vi "HFRR ADV v025 new software.vi"() -> ()   [LabVIEW 2025] (continued)
        n322 = event-data() -> ()  [unwired: 1 in, 6 out]
        n323 = Unbundle By Name("Password 3") -> ("Service Password"=w406:string)
        n324 = call <vilib>:"Trim Whitespace.vi"("string"=w406) -> ("trimmed string"=w404:string)  [unwired: 1 in]
        n325 = Equal?(x=w404, y="Service@123") -> (x = y?=w405:bool)
        n326 = case shown="False" w405 {
          selector: w405 -> [w409 w411]
          frame False {
            n327 = local write "Service Password enable"(w409) -> ()
            n328 = property on="Service Password Log" class="Str"("Visible"=TRUE) -> ()  [unwired: 2 in, 2 out]
          }
          frame True {
            n329 = property on="Service Password Log" class="Str"("Visible"=FALSE) -> ()  [unwired: 2 in, 2 out]
            "Service Password enable" <- w411
          }
        }
      }
      event "Sign In": Value Change {
        w413 = FALSE ("Visible")
        n330 = event-data() -> ()  [unwired: 1 in, 6 out]
        n331 = property on="About" class="Clust (strict)"("Visible"=w413) -> ()  [unwired: 2 in, 2 out]
        n332 = property on="Password 3" class="Clust (strict)"("Visible"=w413) -> ()  [unwired: 2 in, 2 out]
        n333 = property on="Service Password Log" class="Str"("Visible"=FALSE) -> ()  [unwired: 2 in, 2 out]
      }
      event "Info": Value Change {
        n334 = event-data() -> ()  [unwired: 1 in, 6 out]
        n335 = local read "Info"() -> (w415:bool)
        n336 = case shown="False" w415 {
          frame False {
            n337 = property on="About" class="Clust (strict)"("Visible"=FALSE) -> ()  [unwired: 2 in, 2 out]
          }
          frame True {
            n338 = property on="About" class="Clust (strict)"("Visible"=TRUE) -> ()  [unwired: 2 in, 2 out]
          }
        }
      }
      event "Calibration": Value Change {
        n339 = event-data() -> ()  [unwired: 1 in, 6 out]
        n340 = local read "Calibration"() -> (w419:bool)
        n341 = case shown="False" w419 {
          frame False {
            n342 = property on="Calibration 2" class="TabCtl (strict)"("Visible"=FALSE) -> ()  [unwired: 2 in, 2 out]
            n343 = local write "Cal Password"("" ("Cal Password")) -> ()
          }
          frame True {
            n344 = property on="Calibration 2" class="TabCtl (strict)"("Visible"=TRUE) -> ()  [unwired: 2 in, 2 out]
            n345 = local write "Cal Password"("" ("Cal Password")) -> ()
          }
        }
        n346 = property on="Wrong Password" class="Str"("Visible"=FALSE) -> ()  [unwired: 2 in, 2 out]
      }
      event "Cal Password": Value Change {
        n347 = event-data() -> ()  [unwired: 1 in, 6 out]
        n348 = local read "Cal Password"() -> (w427:string)
        n349 = call <vilib>:"Trim Whitespace.vi"("string"=w427) -> ("trimmed string"=w426:string)  [unwired: 1 in]
        n350 = Equal?(x=w426, y="Cal@321") -> (x = y?=w424:bool)
        n351 = case shown="True" w424 {
          frame False {
            n352 = property on="Wrong Password" class="Str"("Visible"=TRUE) -> ()  [unwired: 2 in, 2 out]
          }
          frame True {
            n353 = property on="Wrong Password" class="Str"("Visible"=FALSE) -> ()  [unwired: 2 in, 2 out]
            n354 = local write "Main Tab"(T2."About" ("Main Tab")) -> ()
            n355 = local write "Cal Password"("" ("Cal Password")) -> ()
            n356 = local write "Main Dashboard Buttons"(T1."About" ("Main Dashboard Buttons")) -> ()
            n357 = property on="Calibration 2" class="TabCtl (strict)"("Visible"=FALSE) -> ()  [unwired: 2 in, 2 out]
            n358 = local write "Calibration"(FALSE ("Calibration")) -> ()
          }
        }
      }
      event "Calibration Selection": Value Change {
        n359 = event-data() -> ()  [unwired: 1 in, 6 out]
        n360 = local read "Calibration Selection"() -> (w436:T8)
        n361 = case shown="\"Stroke Calibration\"" w436 {
          tunnel: [T7."Stroke" ("Main Calibration Tab") T7."Friction" ("Main Calibration Tab") T7."Main" ("Main Calibration Tab") T7."Temperature" ("Main Calibration Tab")] -> w435
          frame "Stroke Calibration" {
          }
          frame "Friction Force Calibration" {
          }
          frame Default {
          }
          frame "Temperature Calibration" {
          }
        }
        n362 = local write "Main Calibration Tab"(w435) -> ()
      }
      event "Back Stroke": Value Change {
        n363 = event-data() -> ()  [unwired: 1 in, 6 out]
        n364 = local write "Main Stroke Tab"(T9."Step 1" ("Main Stroke Tab")) -> ()
        n365 = local write "Main Calibration Tab"(T7."Main" ("Main Calibration Tab")) -> ()
        n366 = local write "Back Stroke"(FALSE ("Back Stroke")) -> ()
      }
      event "Step 2 Back": Value Change {
        n367 = event-data() -> ()  [unwired: 1 in, 6 out]
        n368 = local write "Main Stroke Tab"(T9."Step 1" ("Main Stroke Tab")) -> ()
        n369 = local write "Step 2 Back"(FALSE ("Back Stroke")) -> ()
      }
      event "Step 3 Back": Value Change {
        n370 = event-data() -> ()  [unwired: 1 in, 6 out]
        n371 = local write "Main Stroke Tab"(T9."Step 2" ("Main Stroke Tab")) -> ()
        n372 = local write "Step 3 Back"(FALSE ("Back Stroke")) -> ()
      }
      event "Step 4 Back": Value Change {
        n373 = event-data() -> ()  [unwired: 1 in, 6 out]
        n374 = local write "Main Stroke Tab"(T9."Step 3" ("Main Stroke Tab")) -> ()
        n375 = local write "Step 4 Back"(FALSE ("Back Stroke")) -> ()
      }
      event "Step 5 Back": Value Change {
        n376 = event-data() -> ()  [unwired: 1 in, 6 out]
        n377 = local write "Main Stroke Tab"(T9."Step 4" ("Main Stroke Tab")) -> ()
        n378 = local write "Step 5 Back"(FALSE ("Back Stroke")) -> ()
      }
      event "Step 6 Back": Value Change {
        n379 = event-data() -> ()  [unwired: 1 in, 6 out]
        n380 = local write "Main Stroke Tab"(T9."Step 5" ("Main Stroke Tab")) -> ()
        n381 = local write "Step 6 Back"(FALSE ("Back Stroke")) -> ()
      }
      event "Back Stroke step 7": Value Change {
        n382 = event-data() -> ()  [unwired: 1 in, 6 out]
        n383 = local write "Main Stroke Tab"(T9."Step 6" ("Main Stroke Tab")) -> ()
        n384 = local write "Back Stroke step 7"(FALSE ("Back Stroke")) -> ()
      }
      event "Back Stroke step 8": Value Change {
        n385 = event-data() -> ()  [unwired: 1 in, 6 out]
        n386 = local write "Main Stroke Tab"(T9."Step 7" ("Main Stroke Tab")) -> ()
        n387 = local write "Back Stroke step 8"(FALSE ("Back Stroke")) -> ()
      }
      event "Back Stroke 8": Value Change {
        n388 = event-data() -> ()  [unwired: 1 in, 6 out]
        n389 = local write "MOVE CARRIAGE TO"(0.2 ("MOVE CARRIAGE TO")) -> ()
        n390 = local write "Main Stroke Tab"(T9."Step 1" ("Main Stroke Tab")) -> ()
        n391 = local write "Back Stroke 8"(FALSE ("Back Stroke 8")) -> ()
      }
      event "Continue Stroke": Value Change {
        n392 = event-data() -> ()  [unwired: 1 in, 6 out]
        n393 = local write "Main Stroke Tab"(T9."Step 2" ("Main Stroke Tab")) -> ()
        n394 = local write "Continue Stroke"(FALSE ("Continue Stroke")) -> ()
      }
      event "Continue Stroke step 2": Value Change {
        n395 = event-data() -> ()  [unwired: 1 in, 6 out]
        n396 = local write "Main Stroke Tab"(T9."Step 3" ("Main Stroke Tab")) -> ()
        n397 = local write "Continue Stroke step 2"(FALSE ("Continue Stroke")) -> ()
      }
      event "Continue Stroke step 3": Value Change {
        n398 = event-data() -> ()  [unwired: 1 in, 6 out]
        n399 = local write "Main Stroke Tab"(T9."Step 4" ("Main Stroke Tab")) -> ()
        n400 = local write "Continue Stroke step 3"(FALSE ("Continue Stroke")) -> ()
      }
      event "Continue Stroke step 4": Value Change {
        n401 = event-data() -> ()  [unwired: 1 in, 6 out]
        n402 = local write "Main Stroke Tab"(T9."Step 5" ("Main Stroke Tab")) -> ()
        n403 = local write "Continue Stroke step 4"(FALSE ("Continue Stroke")) -> ()
      }
      event "Continue Stroke step 5": Value Change {
        n404 = event-data() -> ()  [unwired: 1 in, 6 out]
        n405 = local write "Main Stroke Tab"(T9."Step 6" ("Main Stroke Tab")) -> ()
        n406 = local write "Continue Stroke step 5"(FALSE ("Continue Stroke")) -> ()
      }
      event "Continue Stroke step 6": Value Change {
        n407 = event-data() -> ()  [unwired: 1 in, 6 out]
        n408 = local write "Main Stroke Tab"(T9."Step 7" ("Main Stroke Tab")) -> ()
        n409 = local write "Continue Stroke step 6"(FALSE ("Continue Stroke")) -> ()
      }
      event "Continue Stroke step 7": Value Change {
        w475 = FALSE ("0.2mm")
        n410 = event-data() -> ()  [unwired: 1 in, 6 out]
        n411 = local write "0.4 mm"(w475) -> ()
        n412 = local write "0.6 mm"(w475) -> ()
        n413 = local write "1.0 mm"(w475) -> ()
        n414 = local write "1.2 mm"(w475) -> ()
        n415 = local write "0.2 2"(w475) -> ()
        n416 = local write "0.4 2"(w475) -> ()
        n417 = local write "0.6 2"(w475) -> ()
        n418 = local write "0.8 2"(w475) -> ()
        n419 = local write "1.0 2"(w475) -> ()
        n420 = local write "1.2"(w475) -> ()
        n421 = local write "0.2mm"(w475) -> ()
        n422 = local write "0.8mm"(w475) -> ()
        n423 = local write "Main Stroke Tab"(T9."Step 8" ("Main Stroke Tab")) -> ()
        n424 = local write "Continue Stroke step 7"(FALSE ("Continue Stroke")) -> ()
        n425 = local write "Stroke Test Complete"(T10."Test Progress" ("Stroke Test Complete")) -> ()
        "Position Measurment Temp" <- 0.0 ("Position Measurment Temp")
        "Calibration Tare" <- TRUE ("Calibration Tare")
        "MOVE CARRIAGE TO" <- 0.2 ("MOVE CARRIAGE TO")
      }
      event "Continue Stroke step 8": Value Change {
        n426 = event-data() -> ()  [unwired: 1 in, 6 out]
        n427 = local read "LVDT STROKE  Calibration"() -> (w480:dbl)
        n428 = local read "Position Measurment Temp"() -> (w481:dbl)
        n429 = case shown="7" w481 {
          selector: w481 -> [w486 w491 w496 w501 w506 w510 w513 w514]
          tunnel: w480 -> [w482 w487 w492 w497 w502 w507 _ _]
          frame 0, Default {
            w484 = TRUE ("0.2mm")
            n430 = Increment(x=w486) -> (x+1=w485:i32)
            n431 = local write "Position Measurment Temp"(w485) -> ()
            n432 = local write "0.2mm"(w484) -> ()
            n433 = local write "0.2 2"(w484) -> ()
            n434 = local write "MOVE CARRIAGE TO"(0.4 ("MOVE CARRIAGE TO")) -> ()
            "Calibration 0.2" <- w482
          }
          frame 1 {
            w489 = TRUE ("0.4 mm")
            n435 = Increment(x=w491) -> (x+1=w490:i32)
            n436 = local write "Calibration 0.4"(w487) -> ()
            n437 = local write "Position Measurment Temp"(w490) -> ()
            n438 = local write "0.4 mm"(w489) -> ()
            n439 = local write "MOVE CARRIAGE TO"(0.6 ("MOVE CARRIAGE TO")) -> ()
            n440 = local write "0.4 2"(w489) -> ()
          }
          frame 2 {
            w494 = TRUE ("0.6 mm")
            n441 = Increment(x=w496) -> (x+1=w495:i32)
            n442 = local write "Calibration 0.6"(w492) -> ()
            n443 = local write "Position Measurment Temp"(w495) -> ()
            n444 = local write "0.6 2"(w494) -> ()
            n445 = local write "0.6 mm"(w494) -> ()
            n446 = local write "MOVE CARRIAGE TO"(0.8 ("MOVE CARRIAGE TO")) -> ()
          }
          frame 3 {
            w498 = TRUE ("0.6 mm")
            n447 = Increment(x=w501) -> (x+1=w500:i32)
            n448 = local write "Position Measurment Temp"(w500) -> ()
            n449 = local write "MOVE CARRIAGE TO"(1.0 ("MOVE CARRIAGE TO")) -> ()
            n450 = local write "0.8mm"(w498) -> ()
            n451 = local write "0.8 2"(w498) -> ()
            "Calibration 0.8" <- w497
          }
          frame 4 {
            w503 = TRUE ("0.6 mm")
            n452 = Increment(x=w506) -> (x+1=w505:i32)
            n453 = local write "Position Measurment Temp"(w505) -> ()
            n454 = local write "MOVE CARRIAGE TO"(1.2 ("MOVE CARRIAGE TO")) -> ()
            n455 = local write "1.0 mm"(w503) -> ()
            n456 = local write "1.0 2"(w503) -> ()
            "Calibration 1.0" <- w502
          }
          frame 5 {
            w508 = TRUE ("0.6 mm")
            n457 = Increment(x=w510) -> (x+1=w509:i32)
            n458 = local write "Position Measurment Temp"(w509) -> ()
            n459 = local write "1.2 mm"(w508) -> ()
            n460 = local write "1.2"(w508) -> ()
            "Calibration 1.2" <- w507
          }
          frame 6 {
            n461 = Increment(x=w513) -> (x+1=w512:i32)
            n462 = local write "Position Measurment Temp"(w512) -> ()
            n463 = local write "Stroke Test Complete"(T10."Stroke Points Completed" ("Stroke Test Complete")) -> ()
          }
          frame 7 {
            n464 = stacked-sequence {
              tunnel: w514 -> [w515 _ _]
              frame #0 {
                n465 = Increment(x=w515) -> (x+1=w516:i32)
                n466 = local write "Main Stroke Tab"(T9."Step 9" ("Main Stroke Tab")) -> ()
                n467 = local write "Position Measurment Temp"(w516) -> ()
                n468 = Insert Into Array(array=dbl[] [], new element #1=0.2 ("new element/subarray"), new element #2=0.4 ("new element/subarray"), new element #3=0.6 ("new element/subarray"), new element #4=0.8 ("new element/subarray"), new element #5=1.0 ("new element/subarray"), new element #6=1.2 ("new element/subarray")) -> (→"1D stroke":dbl[])  [unwired: 1 in]
                n469 = local read "Calibration 0.2"() -> (w523:dbl)
                n470 = local read "Calibration 0.4"() -> (w522:dbl)
                n471 = local read "Calibration 0.6"() -> (w521:dbl)
                n472 = local read "Calibration 0.8"() -> (w520:dbl)
                n473 = local read "Calibration 1.0"() -> (w519:dbl)
                n474 = local read "Calibration 1.2"() -> (w518:dbl)
                n475 = Insert Into Array(array=dbl[] [], new element #1=w523, new element #2=w522, new element #3=w521, new element #4=w520, new element #5=w519, new element #6=w518) -> (→"Calibrated Voltage Value":dbl[])  [unwired: 1 in]
              }
              frame #1 {
                n476 = local read "calibration values"() -> (w546:dbl[])
                n477 = local read "Calibrated Voltage Value"() -> (w548:dbl[])
                n478 = Index Array(array=w546, index #1=1 ("index"), index #2=3 ("index"), index #3=5 ("index"), index #4=7 ("index"), index #5=9 ("index"), index #6=11 ("index")) -> (element #1=w539:dbl, element #2=w538:dbl, element #3=w537:dbl, element #4=w536:dbl, element #5=w535:dbl, element #6=w534:dbl)
                n479 = local read "1D stroke"() -> (w549:dbl[])
                n480 = for {
                  tunnel: [w558] -> w547 mode=indexing
                  tunnel: w549 -> [w557] mode=indexing
                  tunnel: w548 -> [w556] mode=indexing
                  tunnel: w539 -> [w555]
                  tunnel: w538 -> [w554]
                  tunnel: w537 -> [w553]
                  tunnel: w536 -> [w552]
                  tunnel: w535 -> [w551]
                  tunnel: w534 -> [w550]
                  n481 = formula code="if (stroke == 0.2)\n{\n    if ((voltage >= REF_02 * 0.985) && (voltage <= REF_02 * 1.015))\n        status = 1;\n    else\n        status = 0;\n}\nelse if (stroke == 0.4)\n{\n    if ((voltage >= REF_04 * 0.985) && (voltage <= REF_04 * 1.015))\n        status = 1;\n    else\n        status = 0;\n}\nelse if (stroke == 0.6)\n{\n    if ((voltage >= REF_06 * 0.985) && (voltage <= REF_06 * 1.015))\n        status = 1;\n    else\n        status = 0;\n}\nelse if (stroke == 0.8)\n{\n    if ((voltage >= REF_08 * 0.985) && (voltage <= REF_08 * 1.015))\n        status = 1;\n    else\n        status = 0;\n}\nelse if (stroke == 1.0)\n{\n    if ((voltage >= REF_10 * 0.985) && (voltage <= REF_10 * 1.015))\n        status = 1;\n    else\n        status = 0;\n}\nelse if (stroke == 1.2)\n{\n    if ((voltage >= REF_12 * 0.985) && (voltage <= REF_12 * 1.015))\n        status = 1;\n    else\n        status = 0;\n}\nelse\n{\n    status = 0;\n}"("stroke"=w557, "voltage"=w556, "REF_02"=w555, "REF_04"=w554, "REF_06"=w553, "REF_08"=w552, "REF_10"=w551, "REF_12"=w550) -> ("status"=w558:dbl)
                }
                "Status" <- w547
              }
              frame #2 {
                w565 = 1.0
                n482 = local read "Status"() -> (w572:dbl[])
                n483 = Index Array(array=w572) -> (element #1=w571:dbl, element #2=w570:dbl, element #3=w569:dbl, element #4=w568:dbl, element #5=w567:dbl, element #6=w566:dbl)  [unwired: 6 in]
                n484 = Equal?(x=w570, y=w565) -> (x = y?=w563:bool)
                n485 = Equal?(x=w569, y=w565) -> (x = y?=w562:bool)
                n486 = Equal?(x=w568, y=w565) -> (x = y?=w561:bool)
                n487 = Equal?(x=w567, y=w565) -> (x = y?=w560:bool)
                n488 = Equal?(x=w566, y=w565) -> (x = y?=w559:bool)
                n489 = Equal?(x=w571, y=w565) -> (x = y?=w564:bool)
                n490 = case shown="True" w564 {
                  selector: w564 -> [w583 w584]
                  frame True {
                    n491 = local write "Point 1 - 0.2 mm"(w583) -> ()
                    n492 = property on="Point 1 - 0.2 mm" class="Bool"("Caption.Visible"=w583) -> ()  [unwired: 2 in, 2 out]
                  }
                  frame False {
                    n493 = local write "Point 1 - 0.2 mm"(w584) -> ()
                    n494 = property on="Point 1 - 0.2 mm" class="Bool"("Caption.Visible"=w584) -> ()  [unwired: 2 in, 2 out]
                  }
                }
                n495 = case shown="True" w563 {
                  selector: w563 -> [w581 w582]
                  frame True {
                    n496 = local write "Point 2 - 0.4 mm"(w581) -> ()
                    n497 = property on="Point 2 - 0.4 mm" class="Bool"("Caption.Visible"=w581) -> ()  [unwired: 2 in, 2 out]
                  }
                  frame False {
                    n498 = local write "Point 2 - 0.4 mm"(w582) -> ()
                    n499 = property on="Point 2 - 0.4 mm" class="Bool"("Caption.Visible"=w582) -> ()  [unwired: 2 in, 2 out]
                  }
                }
                n500 = case shown="True" w560 {
                  selector: w560 -> [w575 w576]
                  frame True {
                    n501 = local write "Point 5 - 1.0 mm"(w575) -> ()
                    n502 = property on="Point 5 - 1.0 mm" class="Bool"("Caption.Visible"=w575) -> ()  [unwired: 2 in, 2 out]
                  }
                  frame False {
                    n503 = local write "Point 5 - 1.0 mm"(w576) -> ()
                    n504 = property on="Point 5 - 1.0 mm" class="Bool"("Caption.Visible"=w576) -> ()  [unwired: 2 in, 2 out]
                  }
                }
                n505 = case shown="True" w562 {
                  selector: w562 -> [w579 w580]
                  frame True {
                    n506 = local write "Point 3 - 0.6 mm"(w579) -> ()
                    n507 = property on="Point 3 - 0.6 mm" class="Bool"("Caption.Visible"=w579) -> ()  [unwired: 2 in, 2 out]
                  }
                  frame False {
                    n508 = local write "Point 3 - 0.6 mm"(w580) -> ()
                    n509 = property on="Point 3 - 0.6 mm" class="Bool"("Caption.Visible"=w580) -> ()  [unwired: 2 in, 2 out]
                  }
                }
                n510 = case shown="True" w561 {
                  selector: w561 -> [w577 w578]
                  frame True {
                    n511 = local write "Point 4 - 0.8 mm"(w577) -> ()
                    n512 = property on="Point 4 - 0.8 mm" class="Bool"("Caption.Visible"=w577) -> ()  [unwired: 2 in, 2 out]
                  }
                  frame False {
                    n513 = local write "Point 4 - 0.8 mm"(w578) -> ()
                    n514 = property on="Point 4 - 0.8 mm" class="Bool"("Caption.Visible"=w578) -> ()  [unwired: 2 in, 2 out]
                  }
                }
                n515 = case shown="True" w559 {
                  selector: w559 -> [w573 w574]
                  frame True {
                    n516 = local write "Point 6 - 1.2 mm"(w573) -> ()
                    n517 = property on="Point 6 - 1.2 mm" class="Bool"("Caption.Visible"=w573) -> ()  [unwired: 2 in, 2 out]
                  }
                  frame False {
                    n518 = local write "Point 6 - 1.2 mm"(w574) -> ()
                    n519 = property on="Point 6 - 1.2 mm" class="Bool"("Caption.Visible"=w574) -> ()  [unwired: 2 in, 2 out]
                  }
                }
              }
            }
          }
        }
      }
      event "TEMPERATURE STEP Back 1", "TEMPERATURE STEP Back air Temp": Value Change {
        n520 = event-data() -> ()  [unwired: 1 in, 6 out]
        n521 = stacked-sequence {
          frame #0 {
            n522 = local write "Main Calibration Tab"(T7."Main" ("Main Calibration Tab")) -> ()
          }
          frame #1 {
            n523 = Wait (ms)(milliseconds to wait=u32 1000) -> ()  [unwired: 1 out]
          }
          frame #2 {
            n524 = local write "Due Write"("CAL;END" ("Command")) -> ()
          }
          frame #3 {
            n525 = Wait (ms)(milliseconds to wait=u32 2000) -> ()  [unwired: 1 out]
          }
          frame #4 {
            n526 = local write "Due Write"("CAL;END" ("Command")) -> ()
          }
        }
      }
      event "Temperature Continue Step 1": Value Change {
        n527 = event-data() -> ()  [unwired: 1 in, 6 out]
        n528 = stacked-sequence {
          frame #0 {
            n529 = Wait (ms)(milliseconds to wait=u32 1500) -> ()  [unwired: 1 out]
          }
          frame #1 {
            n530 = local write "Due Write"("CAL;START" ("Command")) -> ()
          }
          frame #2 {
            n531 = Wait (ms)(milliseconds to wait=u32 1500) -> ()  [unwired: 1 out]
          }
          frame #3 {
            n532 = local write "Due Write"("CAL;START" ("Command")) -> ()
          }
          frame #4 {
            n533 = Wait (ms)(milliseconds to wait=u32 2000) -> ()  [unwired: 1 out]
          }
          frame #5 {
          }
          frame #6 {
            n534 = Wait (ms)(milliseconds to wait=u32 2000) -> ()  [unwired: 1 out]
          }
          frame #7 {
            # "CAL;A1;<true_T>"
            n535 = local write "Due Write"("CAL;A1;0" ("Command")) -> ()
          }
          frame #8 {
            n536 = local write "Tab Control 4"(T11."Step 2" ("Tab Control 4")) -> ()
          }
        }
      }
      event "Temperature Continue Step air Step 1": Value Change {
        n537 = event-data() -> ()  [unwired: 1 in, 6 out]
        n538 = stacked-sequence {
          frame #0 {
            n539 = Wait (ms)(milliseconds to wait=u32 1500) -> ()  [unwired: 1 out]
          }
          frame #1 {
            n540 = local write "Due Write"("CAL;START" ("Command")) -> ()
          }
          frame #2 {
            n541 = local write "Tab Control 4"(T11."Air Step 2" ("Tab Control 4")) -> ()
            n542 = Wait (ms)(milliseconds to wait=u32 1500) -> ()  [unwired: 1 out]
          }
          frame #3 {
            n543 = local write "Due Write"("CAL;START" ("Command")) -> ()
          }
          frame #4 {
            n544 = Wait (ms)(milliseconds to wait=u32 2000) -> ()  [unwired: 1 out]
          }
          frame #5 {
            # "CAL;A1;<true_T>"
            n545 = local write "Due Write"("CAL;A2;0" ("Command")) -> ()
          }
          frame #6 {
            n546 = Wait (ms)(milliseconds to wait=u32 2000) -> ()  [unwired: 1 out]
          }
          frame #7 {
            # "CAL;A1;<true_T>"
            n547 = local write "Due Write"("CAL;A1;0" ("Command")) -> ()
          }
        }
      }
      event "Temperature Selection": Value Change {
        n548 = event-data() -> ()  [unwired: 1 in, 6 out]
        n549 = local read "Temperature Selection"() -> (w607:enum32{"Air Temperature", "Sample Temperature"})
        n550 = case shown="\"Sample Temperature\"" w607 {
          frame "Air Temperature", Default {
            n551 = local write "Tab Control 4"(T11."Air Step 1" ("Tab Control 4")) -> ()
          }
          frame "Sample Temperature" {
            n552 = local write "Tab Control 4"(T11."Step 1" ("Tab Control 4")) -> ()
          }
        }
      }
      event "Temperature Continue Step 2": Value Change {
        n553 = event-data() -> ()  [unwired: 1 in, 6 out]
        n554 = stacked-sequence {
          frame #0 {
            n555 = stacked-sequence {
              frame #0 {
                n556 = Wait (ms)(milliseconds to wait=u32 1500) -> ()  [unwired: 1 out]
              }
              frame #1 {
                # "CAL;A1;<true_T>"
                n557 = local write "Due Write"("CAL;A1;0" ("Command")) -> ()
              }
              frame #2 {
                n558 = Wait (ms)(milliseconds to wait=u32 1500) -> ()  [unwired: 1 out]
              }
              frame #3 {
                # "CAL;A1;<true_T>"
                n559 = local write "Due Write"("CAL;A1;0" ("Command")) -> ()
              }
              frame #4 {
              }
            }
          }
          frame #1 {
            n560 = local write "Tab Control 4"(T11."Step 3" ("Tab Control 4")) -> ()
          }
        }
      }
      event "Temperature Continue Step 3": Value Change {
        n561 = event-data() -> ()  [unwired: 1 in, 6 out]
        n562 = stacked-sequence {
          frame #0 {
            n563 = stacked-sequence {
              frame #0 {
                n564 = Wait (ms)(milliseconds to wait=u32 1500) -> ()  [unwired: 1 out]
              }
              frame #1 {
              }
              frame #2 {
              }
              frame #3 {
                # "CAL;A1;<true_T>"
                n565 = local write "Due Write"("CAL;A1;60" ("Command")) -> ()
              }
              frame #4 {
                n566 = Wait (ms)(milliseconds to wait=u32 2000) -> ()  [unwired: 1 out]
              }
              frame #5 {
                # "CAL;A1;<true_T>"
                n567 = local write "Due Write"("CAL;A1;60" ("Command")) -> ()
              }
            }
          }
          frame #1 {
            n568 = Wait (ms)(milliseconds to wait=u32 1000) -> ()  [unwired: 1 out]
          }
          frame #2 {
            n569 = local write "Due Write"("CAL;SAVE" ("Command")) -> ()
          }
          frame #3 {
            n570 = Wait (ms)(milliseconds to wait=u32 1000) -> ()  [unwired: 1 out]
          }
          frame #4 {
            n571 = local write "Due Write"("CAL;SAVE" ("Command")) -> ()
          }
          frame #5 {
            n572 = Wait (ms)(milliseconds to wait=u32 1000) -> ()  [unwired: 1 out]
          }
          frame #6 {
            # "CAL;END"
            n573 = local write "Due Write"("CAL;END" ("Command")) -> ()
          }
          frame #7 {
            n574 = Wait (ms)(milliseconds to wait=u32 1000) -> ()  [unwired: 1 out]
          }
          frame #8 {
            # "CAL;END"
            n575 = local write "Due Write"("CAL;END" ("Command")) -> ()
          }
          frame #9 {
            n576 = local write "Main Calibration Tab"(T7."Temperature" ("Main Calibration Tab")) -> ()
            n577 = local write "Tab Control 4"(T11."Main" ("Tab Control 4")) -> ()
          }
        }
      }
      event "Back Stroke step main temperature": Value Change {
        n578 = event-data() -> ()  [unwired: 1 in, 6 out]
        n579 = stacked-sequence {
          frame #0 {
            n580 = Wait (ms)(milliseconds to wait=u32 1000) -> ()  [unwired: 1 out]
          }
          frame #1 {
            # "CAL;END"
            n581 = local write "Due Write"("CAL;END" ("Command")) -> ()
          }
          frame #2 {
            n582 = Wait (ms)(milliseconds to wait=u32 1000) -> ()  [unwired: 1 out]
          }
          frame #3 {
            # "CAL;END"
            n583 = local write "Due Write"("CAL;END" ("Command")) -> ()
          }
          frame #4 {
            n584 = local write "Main Calibration Tab"(T7."Temperature" ("Main Calibration Tab")) -> ()
            n585 = local write "Tab Control 4"(T11."Main" ("Tab Control 4")) -> ()
          }
        }
      }
      event "Quit": Value Change {
        n586 = event-data() -> ()  [unwired: 1 in, 6 out]
      }
    }
    n587 = Wait (ms)(milliseconds to wait=u32 100) -> ()  [unwired: 1 out]
  }
  n588 = while {
    stop <- w640 stop-if-true
    n589 = local read "Ambient Temperature"() -> (w638:dbl)
    n590 = local read "Sample Temperature"() -> (w637:dbl)
    n591 = Wait (ms)(milliseconds to wait=u32 200) -> ()  [unwired: 1 out]
    n592 = local write "Temperature — Live (Set A: 0 °C)"(w638) -> ()
    n593 = local write "Temperature — Live (Set A: 60 °C)"(w638) -> ()
    n594 = local write "Sensor value"(w638) -> ()
    n595 = local write "Sensor value"(w638) -> ()
    n596 = local write "Sensor value"(w637) -> ()
    n597 = local write "Sensor value"(w637) -> ()
    n598 = local write "Temperature — Live (Set A: 60 °C)"(w637) -> ()
    n599 = local write "Temperature — Live (Set A: 60 °C)"(w637) -> ()
    n600 = case shown="True" "Save Button" {
      selector: "Save Button" -> [_ w642]
      frame False {
      }
      frame True {
        n601 = Not(x=w642) -> (.not. x?=w641:bool)
        n602 = local read "milliseconds to wait"() -> (w674:u32)
        n603 = local read "max_step_change"() -> (w679:dbl)
        n604 = local read "max_amplitude"() -> (w680:dbl)
        n605 = local read "min_amplitude"() -> (w681:dbl)
        n606 = local read "PIEZO_CAL_FACTOR"() -> (w685:dbl)
        n607 = local write "Save Button"(w641) -> ()
        n608 = local read "startup_cmd"() -> (w682:dbl)
        n609 = local read "NORMAL_FORCE"() -> (w686:dbl)
        n610 = local read "ADC_Resolution"() -> (w684:dbl)
        n611 = local read "calibration values"() -> (w689:dbl[])
        n612 = local read "kp"() -> (w676:dbl)
        n613 = local read "kd"() -> (w678:dbl)
        n614 = local read "dt"() -> (w675:dbl)
        n615 = local read "ki"() -> (w677:dbl)
        n616 = local read "STROKE FILTER"() -> (w687:i32)
        n617 = local read "Add up Stroke"() -> (w688:dbl)
        n618 = local read "VREF"() -> (w683:dbl)
        n619 = Insert Into Array(array=dbl[] [], new element #1=w674, new element #2=w675, new element #3=w676, new element #4=w677, new element #5=w678, new element #6=w679, new element #7=w680, new element #8=w681, new element #9=w682) -> (w690:dbl[])  [unwired: 1 in]
        n620 = Insert Into Array(array=dbl[] [], new element #1=w683, new element #2=w684, new element #3=w685, new element #4=w686) -> (w691:dbl[])  [unwired: 1 in]
        n621 = Array To Spreadsheet String(delimiter (Tab)=";", array=w689, 3:"" ("format string")) -> (spreadsheet string=w693:string)
        n622 = Insert Into Array(array=dbl[] [], new element #1=w687, new element #2=w688) -> (w692:dbl[])  [unwired: 1 in]
        n623 = call "Write Config.vi"("Stroke Calibration"=w693, "STROKE PARAMETERS"=w692, "ADC PARAMETERS"=w691, "PID  PARAMETERS"=w690) -> ("error out"=w672:errorcluster)  [unwired: 7 in]
        n624 = call "Stall Data Flow.vim"("value in"=w672, "milliseconds to wait"=u32 2000) -> ("value out"=w673:errorcluster)  [unwired: 1 out]
        n625 = call "Read Config.vi"("error in (no error)"=w673) -> ("STROKE PARAMETERS"=w670:dbl[], "ADC PARAMETERS"=w669:dbl[], "PID  PARAMETERS"=w668:dbl[], "Stroke Calibration"=w671:string)  [unwired: 6 in, 1 out]
        n626 = Index Array(array=w668) -> (element #1=w666:dbl, element #2=w665:dbl, element #3=w664:dbl, element #4=w663:dbl, element #5=w662:dbl, element #6=w661:dbl, element #7=w660:dbl, element #8=w659:dbl, element #9=w658:dbl)  [unwired: 9 in]
        n627 = Index Array(array=w669) -> (element #1=w657:dbl, element #2=w656:dbl, element #3=w655:dbl, element #4=w654:dbl)  [unwired: 4 in]
        n628 = Index Array(array=w670) -> (element #1=w653:dbl, element #2=w652:dbl)  [unwired: 2 in]
        n629 = Spreadsheet String To Array(delimiter (Tab)=";", format string="", spreadsheet string=w671, array type (2D Dbl)=dbl[] []) -> (array=w667:dbl[])
        n630 = local write "VREF"(w657) -> ()
        n631 = local write "ADC_Resolution"(w656) -> ()
        n632 = local write "PIEZO_CAL_FACTOR"(w655) -> ()
        n633 = local write "NORMAL_FORCE"(w654) -> ()
        n634 = local write "STROKE FILTER"(w653) -> ()
        n635 = local write "Add up Stroke"(w652) -> ()
        n636 = local write "calibration values"(w667) -> ()
        n637 = local write "milliseconds to wait"(w666) -> ()
        n638 = local write "dt"(w665) -> ()
        n639 = local write "kp"(w664) -> ()
        n640 = local write "ki"(w663) -> ()
        n641 = local write "kd"(w662) -> ()
        n642 = local write "max_step_change"(w661) -> ()
        n643 = local write "max_amplitude"(w660) -> ()
        n644 = local write "min_amplitude"(w659) -> ()
        n645 = local write "startup_cmd"(w658) -> ()
      }
    }
    n646 = local read "Quit"() -> (w640:bool)
  }
  n647 = while {
    shift-right: [w695] -> _
    shift-left: "Enum - Selector" -> [w696]
    stop <- w697 stop-if-true
    # "Auto Start Logic Loop"
    n648 = case shown="\"Humidity & Temperature On\"" w696 {
      tunnel: [w700 w706 w733 w765 w795 Auto_Start_enum."Exit" ("Enum - Selector") Auto_Start_enum."Init" ("Enum - Selector")] -> w695
      frame "Init", Default {
        n649 = local read "Auto Start Test"() -> (w699:bool)
        n650 = Select(t=Auto_Start_enum."Humidity & Temperature On" ("Enum - Selector"), s=w699, f=Auto_Start_enum."Init") -> (s? t:f=w700:T13)
      }
      frame "Humidity & Temperature On" {
        n651 = stacked-sequence {
          tunnel: [_ _ _ _ _ _ Auto_Start_enum."Reach point" ("Enum - Selector")] -> w703
          frame #0 {
            w708 = T17."Disabled and Grayed Out" ("Disabled")
            w709 = TRUE ("Heater Button")
            n652 = property on="Humidity" class="Bool (strict)"("DisabledEnum"=w708) -> ()  [unwired: 2 in, 2 out]
            n653 = property on="Heater Button" class="Bool (strict)"("DisabledEnum"=w708) -> ()  [unwired: 2 in, 2 out]
            n654 = local write "Heater Button"(w709) -> ()
            n655 = local write "Humidity"(w709) -> ()
            n656 = property on="Heater Button" class="Bool (strict)"("Val(Sgnl)"=TRUE ("Value (Signaling)")) -> ()  [unwired: 2 in, 2 out]
          }
          frame #1 {
            n657 = Wait (ms)(milliseconds to wait=u32 3000) -> ()  [unwired: 1 out]
          }
          frame #2 {
            n658 = local read "Set Temp"() -> (w715:dbl)
            n659 = Number To Fractional String(number=w715, precision (6)=i16 2) -> (F-format string=w712:string)  [unwired: 2 in]
            n660 = Concatenate Strings("ST;" ("Command"), w712) -> (w713:string)
            n661 = local write "Due Write"(w713) -> ()
          }
          frame #3 {
            n662 = Wait (ms)(milliseconds to wait=u32 1500) -> ()  [unwired: 1 out]
          }
          frame #4 {
            (unwired) i16 2 ("precision (6)")
            n663 = local read "Write UNO"() -> (w717:string[])
            n664 = local read "Set Rh"() -> (w720:dbl)
            n665 = Number To Fractional String(number=w720) -> (F-format string=w721:string)  [unwired: 3 in]
            n666 = Concatenate Strings("M;" ("new element/subarray"), w721) -> (w722:string)
            n667 = local write "Due Write"("HE;1" ("Command")) -> ()
            n668 = Insert Into Array(array=w717, new element=w722) -> (w718:string[])  [unwired: 1 in]
            n669 = local write "Write UNO"(w718) -> ()
          }
          frame #5 {
            n670 = Wait (ms)(milliseconds to wait=u32 1500) -> ()  [unwired: 1 out]
          }
          frame #6 {
            w725 = TRUE ("Reach point temp")
            n671 = local write "Reach point Humidity"(w725) -> ()
            n672 = local write "Reach point temp"(w725) -> ()
          }
        }
        n673 = local read "Auto Start Test"() -> (w705:bool)
        n674 = Not(x=w705) -> (.not. x?=w704:bool)
        n675 = Select(t=Auto_Start_enum."close", s=w704, f=w703) -> (s? t:f=w706:T13)
      }
      frame "Reach point" {
        w734 = TRUE ("PAUSE")
        w742 = 1.0 ("y")
        w745 = 1.0 ("y")
        n676 = local read "Set Temp"() -> (w727:dbl)
        n677 = local read "Set Humidity:"() -> (w741:dbl)
        n678 = local read "Humidity ( %RH )"() -> (w746:dbl)
        n679 = Add(x=w727, y=w745) -> (x+y=w744:dbl)
        n680 = Subtract(x=w727, y=w745) -> (x-y=w743:dbl)
        n681 = Add(x=w741, y=w742) -> (x+y=w740:dbl)
        n682 = Subtract(x=w741, y=w742) -> (x-y=w739:dbl)
        n683 = local read "TEMP"() -> (w747:dbl)
        n684 = In Range and Coerce(upper limit=w740, x=w746, lower limit=w739) -> (In Range?=w728:bool)  [unwired: 1 out]
        n685 = In Range and Coerce(upper limit=w744, x=w747, lower limit=w743) -> (In Range?=w729:bool)  [unwired: 1 out]
        n686 = case shown="True" w728 {
          frame False {
          }
          frame True {
            n687 = case shown="True" "Reach point Humidity" {
              selector: "Reach point Humidity" -> [_ w753]
              frame False {
              }
              frame True {
                n688 = local read "EVENT LOG"() -> (w750:string)
                n689 = Not(x=w753) -> (.not. x?=w752:bool)
                n690 = local write "Reach point Humidity"(w752) -> ()
                n691 = call "Event Log.vi"("Content"="Target Humidity reached", "EVENT LOG"=w750) -> ("EVENT LOG"=w751:string)  [unwired: 8 in, 1 out]
                n692 = local write "EVENT LOG"(w751) -> ()
              }
            }
          }
        }
        n693 = case shown="True" w729 {
          frame False {
          }
          frame True {
            n694 = case shown="True" "Reach point temp" {
              selector: "Reach point temp" -> [_ w759]
              frame False {
              }
              frame True {
                n695 = local read "EVENT LOG"() -> (w756:string)
                n696 = Not(x=w759) -> (.not. x?=w758:bool)
                n697 = local write "Reach point temp"(w758) -> ()
                n698 = call "Event Log.vi"("Content"="Target Temperature reached", "EVENT LOG"=w756) -> ("EVENT LOG"=w757:string)  [unwired: 8 in, 1 out]
                n699 = local write "EVENT LOG"(w757) -> ()
              }
            }
          }
        }
        n700 = local read "Auto Start Test"() -> (w732:bool)
        n701 = And(x=w729, y=w728) -> (x .and. y?=w738:bool)
        n702 = Select(t=Auto_Start_enum."Maintain Stage" ("Enum - Selector"), s=w738, f=Auto_Start_enum."Reach point" ("Enum - Selector")) -> (s? t:f=w735:T13)
        n703 = Not(x=w732) -> (.not. x?=w731:bool)
        n704 = Select(t=Auto_Start_enum."close", s=w731, f=w735) -> (s? t:f=w733:T13)
        n705 = call "ELAPSED TIMER VI.vi"("RESET"=w734, "PAUSE"=w734) -> ()  [unwired: 7 in, 3 out]
      }
      frame "Maintain Stage" {
        w774 = 2.0 ("y")
        w773 = 1.0 ("y")
        # "Humidity and  temperatures Set Point  have been reached"
        n706 = local read "Set Temp"() -> (w760:dbl)
        n707 = local read "Set Humidity:"() -> (w777:dbl)
        n708 = local read "Humidity ( %RH )"() -> (w780:dbl)
        n709 = Add(x=w760, y=w773) -> (x+y=w779:dbl)
        n710 = Subtract(x=w760, y=w773) -> (x-y=w778:dbl)
        n711 = local read "TEMP"() -> (w781:dbl)
        n712 = Add(x=w777, y=w774) -> (x+y=w776:dbl)
        n713 = Subtract(x=w777, y=w774) -> (x-y=w775:dbl)
        n714 = In Range and Coerce(upper limit=w779, x=w781, lower limit=w778) -> (In Range?=w772:bool)  [unwired: 1 out]
        n715 = In Range and Coerce(upper limit=w776, x=w780, lower limit=w775) -> (In Range?=w771:bool)  [unwired: 1 out]
        n716 = And(x=w772, y=w771) -> (x .and. y?=w770:bool)
        n717 = Not(x=w770) -> (.not. x?=w769:bool)
        n718 = call "ELAPSED TIMER VI.vi"("TARGET"=60.0, "RESET"=w769, "PAUSE"=FALSE) -> ("ELAPSED INDICATION"=w766:bool)  [unwired: 6 in, 2 out]
        n719 = case shown="True" w766 {
          tunnel: w766 -> [_ w784]
          tunnel: [Auto_Start_enum."Maintain Stage" ("Enum - Selector") w783] -> w764
          frame False {
          }
          frame True {
            n720 = stacked-sequence {
              tunnel: w784 -> [_ _ _ _ _]
              tunnel: [_ _ _ _ Auto_Start_enum."Start Stage" ("Enum - Selector")] -> w783
              frame #0 {
                n721 = local read "EVENT LOG"() -> (w786:string)
                n722 = call "Event Log.vi"("Content"="Humidity and temperature set point has stabilized.", "EVENT LOG"=w786) -> ("EVENT LOG"=w787:string)  [unwired: 8 in, 1 out]
                n723 = local write "EVENT LOG"(w787) -> ()
              }
              frame #1 {
                n724 = Wait (ms)(milliseconds to wait=u32 100) -> ()  [unwired: 1 out]
              }
              frame #2 {
                n725 = local read "EVENT LOG"() -> (w790:string)
                n726 = call "Event Log.vi"("Content"="Auto Test Started", "EVENT LOG"=w790) -> ("EVENT LOG"=w791:string)  [unwired: 8 in, 1 out]
                n727 = local write "EVENT LOG"(w791) -> ()
              }
              frame #3 {
                w792 = TRUE ("RUN")
                n728 = local write "RUN"(w792) -> ()
                n729 = property on="Auto Start Temp" class="Bool (strict)"("Val(Sgnl)"=w792) -> ()  [unwired: 2 in, 2 out]
                "Auto Start Temp" <- w792
              }
              frame #4 {
              }
            }
          }
        }
        n730 = local read "Auto Start Test"() -> (w763:bool)
        n731 = Not(x=w763) -> (.not. x?=w762:bool)
        n732 = Select(t=Auto_Start_enum."close", s=w762, f=w764) -> (s? t:f=w765:T13)
      }
      frame "Start Stage" {
        w794 = TRUE ("PAUSE")
        n733 = local read "Auto Start Test"() -> (w799:bool)
        n734 = Not(x=w799) -> (.not. x?=w798:bool)
        n735 = Select(t=Auto_Start_enum."close" ("Enum - Selector"), s=w798, f=Auto_Start_enum."Start Stage" ("Enum - Selector")) -> (s? t:f=w795:T13)
        n736 = call "ELAPSED TIMER VI.vi"("RESET"=w794, "PAUSE"=w794) -> ()  [unwired: 7 in, 3 out]
      }
      frame "close" {
        w801 = FALSE ("Heater Button")
        n737 = local write "RUN"(w801) -> ()
        n738 = local write "Heater Button"(w801) -> ()
        n739 = local write "Humidity"(w801) -> ()
        n740 = local write "Auto Start Test"(w801) -> ()
        n741 = property on="Heater Button" class="Bool (strict)"("Val(Sgnl)"=FALSE ("Value (Signaling)")) -> ()  [unwired: 2 in, 2 out]
      }
      frame "Exit" {
      }
    }
    n742 = Wait (ms)(milliseconds to wait=u32 100) -> ()  [unwired: 1 out]
    n743 = local read "Quit"() -> (w697:bool)
  }
  n744 = property on="Service Password Log" class="Str"("Visible"=w21) -> ()  [unwired: 2 in, 2 out]
  n745 = property on="Password 3" class="Clust (strict)"("Visible"=w21) -> ()  [unwired: 2 in, 2 out]
  n746 = while {
    stop <- w830 stop-if-true
    w813 = errorcluster {"status"=FALSE, "code"=0, "source"=""} ("error in (no error) 3")
    # "this loop is for manual report generation"
    n747 = local read "Confirm Measrurement"() -> (w812:bool)
    n748 = case shown="True" w812 {
      selector: w812 -> [_ w920]
      tunnel: errorcluster {"status"=FALSE, "code"=0, "source"=""} ("error in (no error) 3") -> [_ w921]
      tunnel: [_ w919] -> _
      frame False {
      }
      frame True {
        n749 = stacked-sequence {
          tunnel: w921 -> [_ w954 _]
          tunnel: w920 -> [_ _ w1061]
          tunnel: [_ w942 _] -> w919
          frame #0 {
            n750 = String To Path(string="C:\\LAB-IQ\\Image Calibrate v01.dcf") -> (path=w924:path)
            n751 = Open/Create/Replace File ("Open File")(file path (use dialog)=w924) -> (refnum out=w925:refnum<file>)  [unwired: 5 in, 2 out]
            n752 = for {
              N: 4 -> [_]
              tunnel: w925 -> [w931]
              i -> [w927]
              n753 = Read from Text File ("Read File")(file (use dialog)=w931) -> (text=w932:string)  [unwired: 3 in, 3 out]
              n754 = String Subset(string=w932, offset (0)=6, length (rest)=10 ("length (rest)")) -> (substring=w928:string)
              n755 = Fract/Exp String To Number(string=w928) -> (number=w926:dbl)  [unwired: 3 in, 1 out]
              n756 = case shown="3" w927 {
                tunnel: w926 -> [w933 w934 _ w935 _]
                frame 0 {
                  n757 = local write "5x Gain"(w933) -> ()
                }
                frame 1 {
                  n758 = local write "10x Gain"(w934) -> ()
                }
                frame 2 {
                }
                frame 3 {
                  n759 = local write "100x gain"(w935) -> ()
                }
                frame 4, Default {
                }
              }
            }
          }
          frame #1 {
            n760 = local read "TEST STANDARD"() -> (w937:T3)
            n761 = case shown="\"ISO 12156\"" w937 {
              tunnel: ["ASTM D6079" "ISO 12156"] -> w936
              frame "ASTM D6079", Default {
              }
              frame "ISO 12156" {
              }
            }
            n762 = call "IMAGE ANALYSIS.vi"("Enum"=POST_ANALYSIS_ENUM."GET MEASUREMENTS", "error in"=w954) -> ("error out"=w961:errorcluster)  [unwired: 8 in, 1 out]
            n763 = local read "Magnification :"() -> (w947:string)
            n764 = call "Stall Data Flow.vim"("value in"=w961, "milliseconds to wait"=u32 1000) -> ("value out"=w960:errorcluster)  [unwired: 1 out]
            n765 = local read "Test File List :"() -> (w958:string)
            n766 = case shown="\"10x\"" w947 {
              tunnel: [w997 w998] -> w945
              frame "5x", Default {
                n767 = local read "5x Gain"() -> (w997:dbl)
              }
              frame "10x" {
                # "5x"
                n768 = local read "10x Gain"() -> (w998:dbl)
              }
            }
            n769 = call "IMAGE ANALYSIS.vi"("Enum"=POST_ANALYSIS_ENUM."READ", "error in"=w960) -> ("error out"=w957:errorcluster, "data out"=w948:string)  [unwired: 8 in]
            n770 = Match Pattern(string=w948, regular expression="\"type\": ") -> (after substring=w952:string)  [unwired: 1 in, 3 out]
            n771 = call "IMAGE PATH CREATION PY.vi"("error in (no error)"=w957, "File Name :"=w958) -> ("error out"=w956:errorcluster, "File Path"=w944:path, "File Path String:"=w939:string)  [unwired: 7 in]
            n772 = Match Pattern(string=w952, regular expression=",") -> (before substring=w938:string)  [unwired: 1 in, 3 out]
            n773 = local read "Calibration Tab"() -> (w941:enum32{"Measrument", "Calibrate"})
            n774 = call "Stall Data Flow.vim"("value in"=w956, "milliseconds to wait"=u32 250) -> ("value out"=w940:errorcluster)  [unwired: 1 out]
            n775 = Equal?(x=w938, y="\"rectangle\"") -> (x = y?=w949:bool)
            n776 = case shown="False" w949 {
              tunnel: w948 -> [w1003 w1058]
              tunnel: w945 -> [_ w1049]
              tunnel: cluster{"major":dbl, "minor":dbl, "average":dbl} {"major"=0.0, "minor"=0.0, "average"=0.0} -> [w1001 w1045]
              tunnel: [w1000 w1042] -> w943
              tunnel: w938 -> [w1002 _]
              tunnel: w945 -> [w999 _]
              frame False {
                n777 = Equal?(x=w1002, y="\"line\"") -> (x = y?=w1004:bool)
                n778 = case shown="True" w1004 {
                  tunnel: w1003 -> [_ w1019]
                  tunnel: w1001 -> [w1006 w1018]
                  tunnel: [w1006 w1016] -> w1000
                  tunnel: w999 -> [_ w1015]
                  frame False {
                  }
                  frame True {
                    w1014 = 0.0 ("Major Axis")
                    n779 = Match Pattern(string=w1019, regular expression="\"length_px\":") -> (after substring=w1017:string)  [unwired: 1 in, 3 out]
                    n780 = property on="Major Axis" class="DigNum (strict)"("Caption.Text"="") -> ()  [unwired: 2 in, 2 out]
                    n781 = property on="Minor Axis" class="DigNum (strict)"("Caption.Text"="") -> ()  [unwired: 2 in, 2 out]
                    n782 = property on="Average" class="DigNum (strict)"("Caption.Text"="Line") -> ()  [unwired: 2 in, 2 out]
                    n783 = Fract/Exp String To Number(string=w1017, default (0 dbl)=0.0 ("default (0 DBL)")) -> (number=w1013:dbl)  [unwired: 2 in, 1 out]
                    "Pixel Value" <- w1013
                    n784 = Multiply(x=w1013, y=w1015) -> (x*y=w1026:dbl)
                    n785 = Multiply(x=w1026, y=1000.0) -> (x*y=w1009:dbl)
                    n786 = Divide(x=w1009, y=1000.0) -> (x/y=w1012:dbl)
                    n787 = local write "Measurment (mm)"(w1012) -> ()
                    n788 = Bundle By Name(cluster=w1018, "average"=w1009) -> (w1016:cluster{"major":dbl, "minor":dbl, "average":dbl})
                    n789 = Number To Fractional String(number=w1009, precision (6)=i16 1) -> (F-format string=w1008:string)  [unwired: 2 in]
                    n790 = local write "Minor Axis"(w1014) -> ()
                    n791 = local write "Major Axis"(w1014) -> ()
                    n792 = Fract/Exp String To Number(string=w1008) -> (number=w1007:dbl)  [unwired: 3 in, 1 out]
                    n793 = local write "Average"(w1007) -> ()
                  }
                }
              }
              frame True {
                w1046 = 1000.0 ("y")
                w1052 = 0.0 ("default (0 DBL)")
                n794 = Match Pattern(string=w1058, regular expression=" \"width_px\":") -> (after substring=w1056:string)  [unwired: 1 in, 3 out]
                n795 = Match Pattern(string=w1056, regular expression="\"height_px\":") -> (before substring=w1054:string, after substring=w1053:string)  [unwired: 1 in, 2 out]
                n796 = Fract/Exp String To Number(string=w1054, default (0 dbl)=w1052) -> (number=w1051:dbl)  [unwired: 2 in, 1 out]
                n797 = Fract/Exp String To Number(string=w1053, default (0 dbl)=w1052) -> (number=w1050:dbl)  [unwired: 2 in, 1 out]
                n798 = Multiply(x=w1051, y=w1049) -> (x*y=w1048:dbl)
                n799 = Multiply(x=w1050, y=w1049) -> (x*y=w1047:dbl)
                n800 = Multiply(x=w1048, y=w1046) -> (x*y=w1032:dbl)
                n801 = Multiply(x=w1047, y=w1046) -> (x*y=w1030:dbl)
                n802 = Add(x=w1032, y=w1030) -> (x+y=w1044:dbl)
                n803 = property on="Major Axis" class="DigNum (strict)"("Caption.Text"="Major Axis") -> ()  [unwired: 2 in, 2 out]
                n804 = property on="Minor Axis" class="DigNum (strict)"("Caption.Text"="Minor Axis") -> ()  [unwired: 2 in, 2 out]
                n805 = property on="Average" class="DigNum (strict)"("Caption.Text"="Average") -> ()  [unwired: 2 in, 2 out]
                n806 = Divide(x=w1044, y=2.0) -> (x/y=w1028:dbl)
                n807 = Bundle By Name(cluster=w1045, "major"=w1032, "minor"=w1030, "average"=w1028) -> (w1042:cluster{"major":dbl, "minor":dbl, "average":dbl})
                n808 = Number To Fractional String(number=w1030, precision (6)=i16 1) -> (F-format string=w1037:string)  [unwired: 2 in]
                n809 = Number To Fractional String(number=w1028, precision (6)=i16 1) -> (F-format string=w1038:string)  [unwired: 2 in]
                n810 = Number To Fractional String(number=w1032, precision (6)=i16 1) -> (F-format string=w1036:string)  [unwired: 2 in]
                n811 = Fract/Exp String To Number(string=w1037) -> (number=w1029:dbl)  [unwired: 3 in, 1 out]
                n812 = Fract/Exp String To Number(string=w1038) -> (number=w1027:dbl)  [unwired: 3 in, 1 out]
                n813 = Fract/Exp String To Number(string=w1036) -> (number=w1031:dbl)  [unwired: 3 in, 1 out]
                n814 = local write "Major Axis"(w1031) -> ()
                n815 = local write "Average"(w1027) -> ()
                n816 = local write "Minor Axis"(w1029) -> ()
              }
            }
            n817 = case shown="\"Measrument\", Default" w941 {
              tunnel: w944 -> [w971 _]
              tunnel: w943 -> [w970 _]
              tunnel: [w967 w996] -> w942
              tunnel: w940 -> [w969 w996]
              tunnel: w939 -> [w968 _]
              tunnel: w936 -> [w966 _]
              frame "Measrument", Default {
                n818 = stacked-sequence {
                  tunnel: w971 -> [w989 _]
                  tunnel: w970 -> [w987 _]
                  tunnel: w969 -> [w985 _]
                  tunnel: w968 -> [w984 _]
                  tunnel: [w979 _] -> w967
                  tunnel: w966 -> [w972 _]
                  frame #0 {
                    n819 = call "IMAGE ANALYSIS.vi"("Enum"=POST_ANALYSIS_ENUM."SAVE IMAGE", "error in"=w985, "IMAGE FILE PATH"=w984) -> ("error out"=w983:errorcluster)  [unwired: 7 in, 1 out]
                    n820 = call "Stall Data Flow.vim"("value in"=w983, "milliseconds to wait"=u32 1000) -> ("value out"=w974:errorcluster)  [unwired: 1 out]
                    n821 = local read "Test File List :"() -> (w991:string)
                    n822 = call "IMAGE ANALYSIS.vi"("Enum"=POST_ANALYSIS_ENUM."MINIMIZE UI", "error in"=w974) -> ("error out"=w981:errorcluster)  [unwired: 8 in, 1 out]
                    n823 = Bundle By Name(cluster=T23 {"File Name"="", "Test Method"="", "Operator"="", "Fuel Description"="", "Date and time"=""} ("Main Ref"), "Test Method"=w972, "File Name"=w991) -> (w992:T23)
                    n824 = call "Stall Data Flow.vim"("value in"=w981, "milliseconds to wait"=u32 1500) -> ("value out"=w976:errorcluster)  [unwired: 1 out]
                    n825 = call "duf file read.vi"("error in (no error)"=w976, "Main Ref"=w992) -> ("error out"=w990:errorcluster, "Main Ref 2"=w988:T23)  [unwired: 8 in]
                    n826 = call "DETECTION REPORT for manual.vi"("error in (no error)"=w990, "return value 3"=w987, "Image File Path"=w989, "Main Ref"=w988) -> ("error out"=w986:errorcluster)  [unwired: 7 in]
                    n827 = call <vilib>:"Clear Errors.vi"("error in (no error)"=w986) -> ("error out"=w977:errorcluster)  [unwired: 5 in, 1 out]
                    n828 = call "IMAGE ANALYSIS.vi"("Enum"=POST_ANALYSIS_ENUM."MINIMIZE UI", "error in"=w977) -> ("error out"=w979:errorcluster)  [unwired: 8 in, 1 out]
                  }
                  frame #1 {
                    n829 = local write "Main Tab"(T2."HOME" ("Main Tab")) -> ()
                    n830 = local write "Main Dashboard Buttons"(T1."Home" ("Main Dashboard Buttons")) -> ()
                  }
                }
              }
              frame "Calibrate" {
              }
            }
          }
          frame #2 {
            n831 = Not(x=w1061) -> (.not. x?=w1060:bool)
            n832 = local write "Confirm Measrurement"(w1060) -> ()
            n833 = local read "Calibration Tab"() -> (w1059:enum32{"Measrument", "Calibrate"})
            n834 = case shown="\"Measrument\", Default" w1059 {
              frame "Measrument", Default {
                (unwired) T18."HOME" ("Main Tab")
                n835 = local write "Main Tab"(T2."HOME" ("Main Tab")) -> ()
              }
              frame "Calibrate" {
              }
            }
          }
        }
      }
    }
    n836 = local read "Humidity"() -> (w804:bool)
    n837 = local read "Save Change"() -> (w809:bool)
    n838 = local read "Calibrate"() -> (w810:bool)
    n839 = local read "Auto Start Test"() -> (w805:bool)
    n840 = case shown="True" w810 {
      selector: w810 -> [_ w917]
      frame False {
      }
      frame True {
        n841 = Not(x=w917) -> (.not. x?=w916:bool)
        n842 = local write "Calibrate"(w916) -> ()
        n843 = local write "Calibration Tab"(enum32{"Measrument", "Calibrate"}."Calibrate" ("Calibration Tab")) -> ()
      }
    }
    n844 = case shown="True" w809 {
      selector: w809 -> [_ w861]
      frame False {
      }
      frame True {
        n845 = stacked-sequence {
          tunnel: w861 -> [_ _ _ _ w915]
          frame #0 {
            n846 = call "IMAGE ANALYSIS.vi"("Enum"=POST_ANALYSIS_ENUM."HIDE UI") -> ()  [unwired: 9 in, 2 out]
          }
          frame #1 {
            n847 = local read "100x gain"() -> (w863:dbl)
            n848 = local read "10x Gain"() -> (w864:dbl)
            n849 = local read "5x Gain"() -> (w865:dbl)
            n850 = Number To Fractional String(number=w864, width (-)=i16 4, precision (6)=i16 7) -> (F-format string=w886:string)  [unwired: 1 in]
            n851 = Number To Fractional String(number=0.0, width (-)=i16 4, precision (6)=i16 7) -> (F-format string=w881:string)  [unwired: 1 in]
            n852 = Number To Fractional String(number=w863, width (-)=i16 4, precision (6)=i16 7) -> (F-format string=w869:string)  [unwired: 1 in]
            n853 = Number To Fractional String(number=w865, width (-)=i16 10 ("precision (6)"), precision (6)=i16 7) -> (F-format string=w895:string)  [unwired: 1 in]
            n854 = Concatenate Strings("[CH1]" ("string"), w895, " - 5x Gain" ("string"), "\r") -> (w885:string)
            n855 = Concatenate Strings("[CH2]" ("string"), w886, " - 10x Gain" ("string"), "\r") -> (w884:string)
            n856 = Concatenate Strings("[CH3]" ("string"), w881, " - 20x Gain" ("string"), "\r") -> (w875:string)
            n857 = Concatenate Strings("[CH4]" ("string"), w869, " - 100x Gain" ("string"), "\r") -> (w868:string)
            n858 = String To Path(string="C:\\LAB-IQ\\Image Calibrate v01.dcf") -> (path=w898:path)
            n859 = Concatenate Strings(w885, w884, w875, w868) -> (w883:string)
            n860 = call <vilib>:"Write Characters To File.vi"("append to file? (new file:F)"=FALSE, "character string"=w883, "file path (dialog if empty)"=w898) -> ()  [unwired: 2 in, 1 out]
          }
          frame #2 {
            n861 = String To Path(string="C:\\LAB-IQ\\Image Calibrate v01.dcf") -> (path=w901:path)
            n862 = Open/Create/Replace File ("Open File")(file path (use dialog)=w901) -> (refnum out=w902:refnum<file>)  [unwired: 5 in, 2 out]
            n863 = for {
              N: 4 -> [_]
              tunnel: w902 -> [w908]
              i -> [w904]
              n864 = Read from Text File ("Read File")(file (use dialog)=w908) -> (text=w909:string)  [unwired: 3 in, 3 out]
              n865 = String Subset(string=w909, offset (0)=6, length (rest)=10 ("length (rest)")) -> (substring=w905:string)
              n866 = Fract/Exp String To Number(string=w905) -> (number=w903:dbl)  [unwired: 3 in, 1 out]
              n867 = case shown="3" w904 {
                tunnel: w903 -> [w910 w911 _ w912 _]
                frame 0 {
                  n868 = local write "5x Gain"(w910) -> ()
                }
                frame 1 {
                  n869 = local write "10x Gain"(w911) -> ()
                }
                frame 2 {
                }
                frame 3 {
                  n870 = local write "100x gain"(w912) -> ()
                }
                frame 4, Default {
                }
              }
            }
          }
          frame #3 {
            n871 = call "IMAGE ANALYSIS.vi"("Enum"=POST_ANALYSIS_ENUM."SHOW UI") -> ()  [unwired: 9 in, 2 out]
          }
          frame #4 {
            n872 = Not(x=w915) -> (.not. x?=w914:bool)
            n873 = local write "Save Change"(w914) -> ()
          }
        }
      }
    }
    n874 = case shown="False" w805 {
      tunnel: w804 -> [w831 _]
      frame False {
        n875 = case shown="True" w831 {
          frame False {
          }
          frame True {
            n876 = local read "Set Humidity:"() -> (w835:dbl)
            n877 = local read "Set Humidity:"() -> (w838:dbl)
            n878 = local read "Humidity ( %RH )"() -> (w839:dbl)
            n879 = Subtract(x=w835, y=2.0) -> (x-y=w833:dbl)
            n880 = Add(x=w838, y=2.0) -> (x+y=w834:dbl)
            n881 = In Range and Coerce(upper limit=w834, x=w839, lower limit=w833) -> (In Range?=w832:bool)  [unwired: 1 out]
            n882 = case shown="True" w832 {
              frame False {
              }
              frame True {
                n883 = case shown="True" "Manual Humididty Reached" {
                  selector: "Manual Humididty Reached" -> [_ w842]
                  frame False {
                  }
                  frame True {
                    n884 = Not(x=w842) -> (.not. x?=w841:bool)
                    n885 = local write "Manual Humididty Reached"(w841) -> ()
                    n886 = local read "EVENT LOG"() -> (w844:string)
                    n887 = call "Event Log.vi"("Content"="Target Humidity reached", "EVENT LOG"=w844) -> ("EVENT LOG"=w843:string)  [unwired: 8 in, 1 out]
                    n888 = local write "EVENT LOG"(w843) -> ()
                  }
                }
              }
            }
          }
        }
      }
      frame True {
        n889 = local write "Manual Humididty Reached"(TRUE ("Manual Humididty Reached")) -> ()
      }
    }
    n890 = local read "Cap Live Image"() -> (w825:bool)
    n891 = local read "SCAR MEASURMENT"() -> (w828:enum32{"Auto Scar", "Manual Scar"})
    n892 = Wait (ms)(milliseconds to wait=u32 250) -> ()  [unwired: 1 out]
    n893 = Equal?(x=w828, y=enum32{"Auto Scar", "Manual Scar"}."Manual Scar" ("SCAR MEASURMENT")) -> (x = y?=w826:bool)
    n894 = And(x=w826, y=w825) -> (x .and. y?=w824:bool)
    n895 = case shown="True" w824 {
      selector: w824 -> [_ w1140]
      frame False {
      }
      frame True {
        n896 = stacked-sequence {
          tunnel: [_ _ _ w1155 _] -> _
          tunnel: w1140 -> [_ _ _ _ w1162]
          frame #0 {
            w1141 = 0.0
            n897 = local write "Major Axis"(w1141) -> ()
            n898 = local write "Minor Axis"(w1141) -> ()
            n899 = local write "Average"(w1141) -> ()
          }
          frame #1 {
            n900 = call "CAMERA LIVE FEED FGV.vi"("Enum - Menu"=CAMERA_LIVE_FEED_ENUM."CAMERA MINIMIZE") -> ()  [unwired: 9 in, 2 out]
          }
          frame #2 {
            n901 = local read "FILE 3"() -> (w1149:string)
